vi "teleop.vi"   [LabVIEW 2010, in "LASA Beta.lvrbt"]
uses:
  LASA Beta.lvrbt
  op_init.vi
  <vilib>/NXT/Dual Mode Library/Display/drawText.vi
  op_run.vi
  <vilib>/NXT/Dual Mode Library/prims/inRangeAndCoerce/inRangeAndCoerce_float.vi
types:
  T1 = typedef "LVHSConnector.ctl" = cluster{"Hardware":string, "Flattened String":string}
  T2 = typedef "FTC ControllerState.ctl" = cluster{"Left X":i8, "Left Y":i8, "Right X":i8, "Right Y":i8, "Button Encoding 9-12":u8, "Button Encoding 1-8":u8, "POV":T3}
  T3 = typedef "FTC POVState.ctl" = i8
  T4 = typedef "FTC ButtonState.ctl" = cluster{"Button 1":bool, "Button 2":bool, "Button 3":bool, "Button 4":bool, "Button 5":bool, "Button 6":bool, "Button 7":bool, "Button 8":bool, "Button 9":bool, "Button 10":bool, "Button 11":bool, "Button 12":bool, "POV":T3}
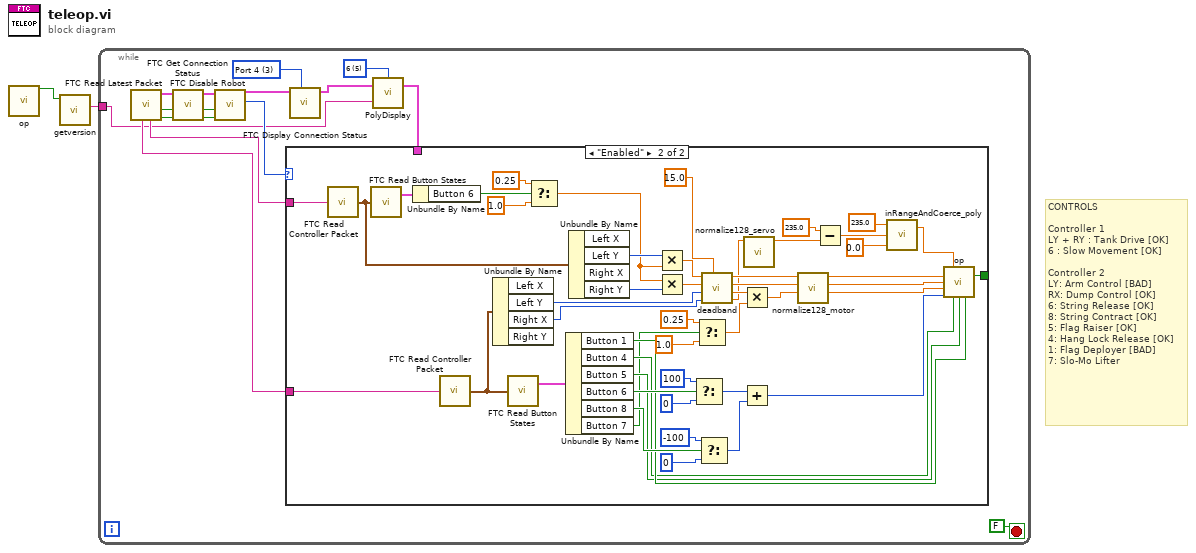
[diagram p0: block diagram]
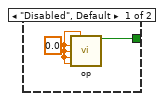
[diagram p2: hidden frame]
diagram:
  # "CONTROLS\n\nController 1\nLY + RY : Tank Drive [OK]\n6 : Slow Movement [OK]\n\nController 2\nLY: Arm Control [BAD]\nRX: Dump Control [OK]\n6: String Release [OK]\n8: String Contract [OK]\n5: Flag Raiser [OK]\n4: Hang Lock Release [OK]\n1: Flag Deployer [BAD]\n7: Slo-Mo Lifter"
  n1 = call-poly "op.vi"() -> ("Chain OUT"=w2:bool)  [unwired: 15 in]
  n2 = call "getversion.vi"("Chain IN"=w2) -> ("Version"=w1:string)  [unwired: 9 in, 1 out]
  n3 = while {
    tunnel: w1 -> [w4]
    stop <- FALSE stop-if-true
    w5 = i16 5 items=["1", "2", "3", "4", "5", "6", "7", "8"] ("Line")
    w7 = u8 3 items=["Port 1", "Port 2", "Port 3", "Port 4"] ("Port")
    n4 = call <vilib>:"FTC Read Latest Packet.vi"() -> ("Packet Received?"=w18:bool, "Stopped?"=w16:bool, "NXT"=w17:T1, "Controller 1"=w13:string, "Controller 2"=w9:string)  [unwired: 6 in, 1 out]
    n5 = call <vilib>:"FTC Get Connection Status.vi"("Packet Received?"=w18, "Stopped?"=w16, "NXT"=w17) -> ("Online?"=w14:bool, "Stopped?"=w15:bool, "NXT"=w11:T1)  [unwired: 5 in]
    n6 = call <vilib>:"FTC Disable Robot.vi"("Online?"=w14, "Stopped?"=w15, "NXT"=w11) -> ("Enabled?"=w12:enum16{"Disabled", "Enabled"}, "NXT"=w8:T1)  [unwired: 3 in]
    n7 = call <vilib>:"FTC Display Connection Status.vi"("Port"=w7, "NXT"=w8) -> ("NXT"=w6:T1)  [unwired: 9 in]
    n8 = call-poly <vilib>:"PolyDisplay.vi"("Text"=w4, "NXT"=w6, "Line"=w5) -> ("NXT"=w3:T1)  [unwired: 1 in]
    n9 = case shown="\"Enabled\"" w12 {
      tunnel: w13 -> [_ w68]
      tunnel: w9 -> [_ w67]
      tunnel: [w19 w21] -> _
      tunnel: w3 -> [_ _]
      frame "Disabled", Default {
        w20 = 0.0 ("Left Drive")
        n10 = call-poly "op.vi"("Dump Control"=w20, "Left Drive"=w20, "Right Drive"=w20, "Arm Control"=w20, "Lift String Control"=w20) -> ("Chain OUT"=w19:bool)  [unwired: 10 in]
      }
      frame "Enabled" {
        n11 = call <vilib>:"FTC Read Controller Packet.vi"("Packet"=w68) -> ("Controller State"=w65:T2)  [unwired: 4 in]
        n12 = call <vilib>:"FTC Read Button States.vi"("Controller State"=w65) -> ("Button States"=w64:T4)  [unwired: 2 in, 1 out]
        n13 = Unbundle By Name(w64) -> ("Button 6"=w32:bool)
        n14 = call <vilib>:"FTC Read Controller Packet.vi"("Packet"=w67) -> ("Controller State"=w66:T2)  [unwired: 4 in]
        n15 = Unbundle By Name(w66) -> ("Left Y"=w49:i8, "Right X"=w47:i8)  [unwired: 2 out]
        n16 = call <vilib>:"FTC Read Button States.vi"("Controller State"=w66) -> ("Button States"=w62:T4)  [unwired: 2 in, 1 out]
        n17 = Select(t=0.25, s=w32, f=1.0) -> (s? t:f=w29:dbl)
        n18 = Unbundle By Name(w62) -> ("Button 1"=w38:bool, "Button 4"=w34:bool, "Button 5"=w33:bool, "Button 6"=w61:bool, "Button 8"=w56:bool, "Button 7"=w25:bool)
        n19 = Unbundle By Name(w65) -> ("Left Y"=w39:i8, "Right Y"=w40:i8)  [unwired: 2 out]
        n20 = Multiply(x=w39, y=w29) -> (x*y=w53:dbl)
        n21 = Multiply(x=w29, y=w40) -> (x*y=w52:dbl)
        n22 = Select(t=100, s=w61, f=0) -> (s? t:f=w55:i32)
        n23 = Select(t=0.25, s=w25, f=1.0) -> (s? t:f=w22:dbl)
        n24 = Select(t=-100, s=w56, f=0) -> (s? t:f=w54:i32)
        n25 = call "deadband.vi"("Deadband"=15.0, "D"=w47, "C"=w49, "B"=w52, "A"=w53) -> ("mD"=w45:dbl, "mC"=w48:dbl, "mB"=w50:dbl, "mA"=w51:dbl)
        n26 = Multiply(x=w48, y=w22) -> (x*y=w26:dbl)
        n27 = Add(x=w55, y=w54) -> (x+y=w35:i32)
        n28 = call "normalize128_servo.vi"("A"=w45) -> ("mA"=w44:dbl)  [unwired: 3 in, 3 out]
        n29 = call "normalize128_motor.vi"("C"=w26, "B"=w50, "A"=w51) -> ("mC"=w37:dbl, "mB"=w27:dbl, "mA"=w28:dbl)  [unwired: 1 in, 1 out]
        n30 = Subtract(x=235.0, y=w44) -> (x-y=w43:dbl)
        n31 = call-poly <vilib>:"inRangeAndCoerce_poly.vi"("lower limit"=0.0, "x"=w43, "upper limit"=235.0) -> ("coerced(x)"=w36:dbl)  [unwired: 1 out]
        n32 = call-poly "op.vi"("Dump Control"=w36, "Left Drive"=w28, "Right Drive"=w27, "Arm Control"=w37, "Lift String Control"=w35, "Release Hang Lock"=w34, "Flag Raiser"=w33, "Flag Deployer"=w38) -> ("Chain OUT"=w21:bool)  [unwired: 7 in]
      }
    }
  }
